vi "IncrementGetVersionSerializable.vi"(4 "SerializableData_v2.ctl":path, 6 "GetVersionSerializableData.vi":path, 7 "New BlueSerializableVersion":u16, 8 "error in (no error)":errorcluster, 10 "Application":refnum<vi>, 11 "LVClassLibrary Ref":refnum<vi>) -> (0 "error out":errorcluster, 2 "Application":refnum<vi>, 3 "LVClassLibrary Ref":refnum<vi>)   [LabVIEW 2019, in "BlueSerializationScripts.lvlib"]
uses:
  BlueSerializationScripts.lvlib
  c2c98d73-d560-4284-ae97-d7d7fd823281.vi
  <vilib>/Utility/error.llb/Clear Errors.vi
  BlueSerialProviderGlobal.vi
  <vilib>/Utility/traverseref.llb/Traverse for GObjects.vi
  BlueUtilityScripts/RefIsOwner.vi
  BlueUtilityScripts/BlueUtilityScripts.lvlib
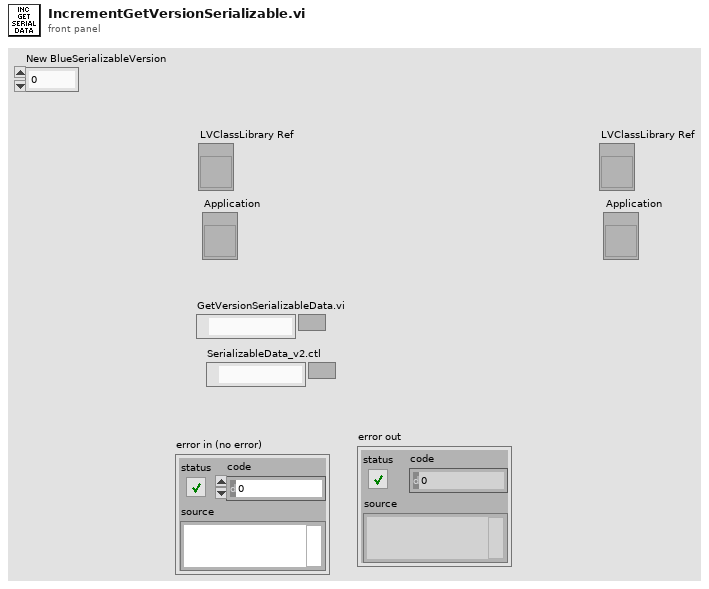
[diagram p1: front panel]
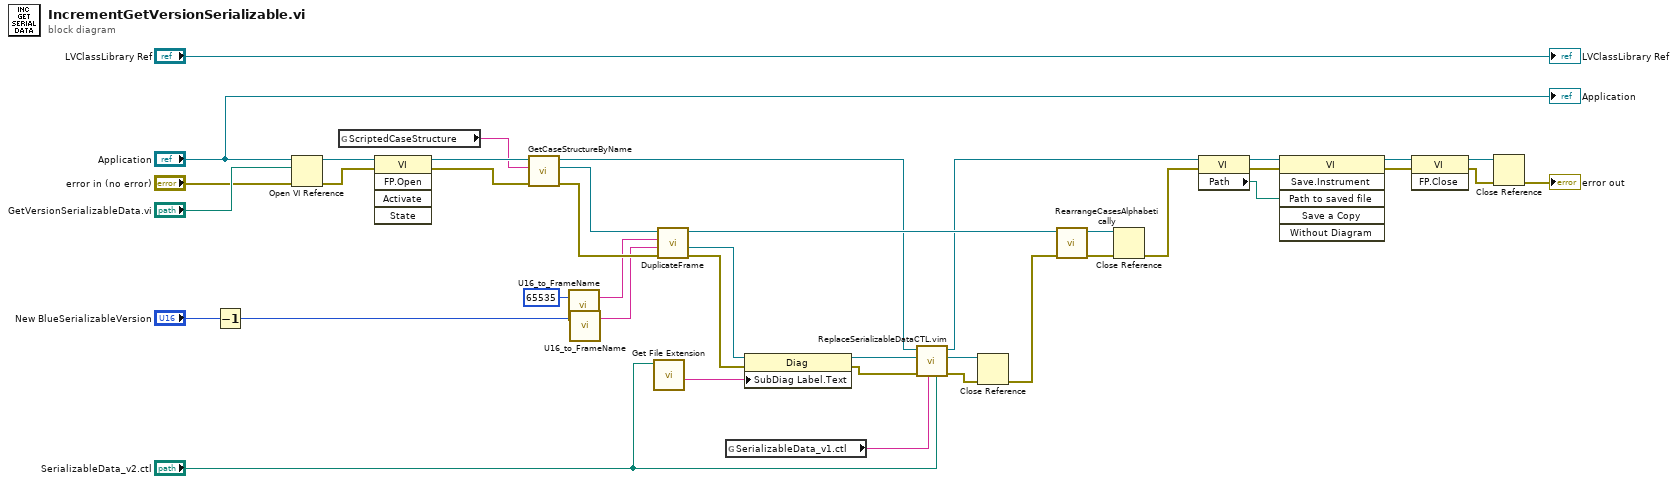
[diagram p0: block diagram]
diagram:
  n1 = Decrement(x="New BlueSerializableVersion") -> (x-1=w17:u16)
  n2 = Open VI Reference(application reference (local)="Application", vi path="GetVersionSerializableData.vi", error in (no error)="error in (no error)") -> (vi reference=w32:refnum<vi>, error out=w31:errorcluster)  [unwired: 3 in]
  n3 = global read "BlueSerialProviderGlobal.vi" "ScriptedCaseStructure"() -> (w27:string)
  n4 = invoke class="VI" method="FP.Open"(reference=w32, error in=w31) -> (reference out=w28:refnum<vi>, error out=w26:errorcluster)  [unwired: 3 in, 3 out]
  n5 = call "GetCaseStructureByName.vi"("error in (no error)"=w26, "CaseStructureLabel.Text"=w27, "VI Refnum"=w28) -> ("error out"=w21:errorcluster, "CaseStructure Ref"=w25:refnum<vi>, "VI Refnum"=w3:refnum<vi>)  [unwired: 6 in]
  n6 = call "U16_to_FrameName.vi"("u16"=u16 65535) -> ("FrameName"=w19:string)  [unwired: 2 in]
  n7 = call "U16_to_FrameName.vi"("u16"=w17) -> ("FrameName"=w18:string)  [unwired: 2 in]
  n8 = call <vilib>:"Get File Extension.vi"("file"="SerializableData_v2.ctl") -> ("filename without extension"=w8:string)  [unwired: 6 in, 4 out]
  n9 = call "DuplicateFrame.vi"("error in (no error)"=w21, "New FrameName"=w18, "FrameName to duplicate"=w19, "CaseStructure Ref"=w25) -> ("error out"=w15:errorcluster, "New Frame"=w16:refnum<vi>, "CaseStructure Ref"=w24:refnum<vi>)  [unwired: 5 in]
  n10 = global read "BlueSerialProviderGlobal.vi" "SerializableData_v1.ctl"() -> (w5:string)
  n11 = property class="Diag"(reference=w16, error in=w15, "SubDiag Label.Text"=w8) -> (reference out=w7:refnum<vi>, error out=w6:errorcluster)
  n12 = call "ReplaceSerializableDataCTL.vim"("CTL path"="SerializableData_v2.ctl", "TypedefPath Name"=w5, "error in (no error)"=w6, "Owner"=w7, "VI Refnum"=w3) -> ("error out"=w14:errorcluster, "dup Owner"=w1:refnum<vi>, "dup VI Refnum"=w2:refnum<vi>)  [unwired: 4 in]
  n13 = Close Reference(reference=w1, error in (no error)=w14) -> (error out=w13:errorcluster)
  n14 = call "RearrangeCasesAlphabetically.vi"("error in (no error)"=w13, "CaseStructure Ref"=w24) -> ("error out"=w22:errorcluster, "CaseStructure Ref"=w23:refnum<vi>)  [unwired: 8 in]
  n15 = Close Reference(reference=w23, error in (no error)=w22) -> (error out=w11:errorcluster)
  n16 = property class="VI"(reference=w2, error in=w11) -> (reference out=w12:refnum<vi>, error out=w9:errorcluster, "Path"=w10:path)
  n17 = invoke class="VI" method="Save.Instrument"(reference=w12, error in=w9, "Path to saved file"=w10) -> (reference out=w40:refnum<vi>, error out=w39:errorcluster)  [unwired: 3 in, 4 out]
  n18 = invoke class="VI" method="FP.Close"(reference=w40, error in=w39) -> (reference out=w38:refnum<vi>, error out=w37:errorcluster)  [unwired: 1 in, 1 out]
  n19 = Close Reference(reference=w38, error in (no error)=w37) -> (error out=→"error out":errorcluster)
  "LVClassLibrary Ref" <- "LVClassLibrary Ref"
  "Application" <- "Application"
